vi "TempControlLoop.vi"(3 "Duty Cycle [0-100%]":dbl, 4 "Period [ms]":dbl, 5 "Count in":u32) -> (1 "State":bool, 2 "Count out":u32)   [LabVIEW 2020]
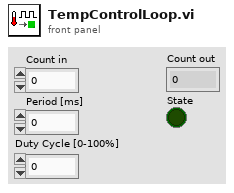
[diagram p1: front panel]
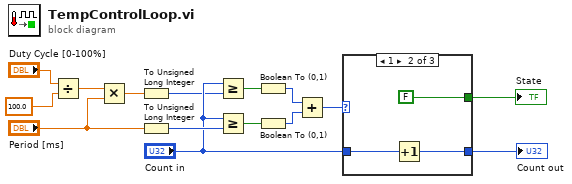
[diagram p0: block diagram]
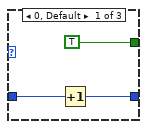
[diagram p2: hidden frame]
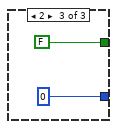
[diagram p3: hidden frame]
diagram:
  n1 = Divide(x="Duty Cycle [0-100%]", y=100.0) -> (x/y=w3:dbl)
  n2 = Multiply(x=w3, y="Period [ms]") -> (x*y=w4:dbl)
  n3 = To Unsigned Long Integer(number=w4) -> (unsigned 32bit integer=w6:u32)
  n4 = To Unsigned Long Integer(number="Period [ms]") -> (unsigned 32bit integer=w15:u32)
  n5 = Greater Or Equal?(x="Count in", y=w6) -> (x >= y?=w7:bool)
  n6 = Greater Or Equal?(x="Count in", y=w15) -> (x >= y?=w8:bool)
  n7 = Boolean To (0,1)(Boolean=w7) -> (0, 1=w9:i16)
  n8 = Boolean To (0,1)(Boolean=w8) -> (0, 1=w10:i16)
  n9 = Add(x=w9, y=w10) -> (x+y=w11:i16)
  n10 = case shown="1" w11 {
    tunnel: "Count in" -> [w18 w21 _]
    tunnel: [w17 w20 u32 0] -> w13
    tunnel: [TRUE FALSE FALSE] -> w14
    frame 0, Default {
      n11 = Increment(x=w18) -> (x+1=w17:u32)
    }
    frame 1 {
      n12 = Increment(x=w21) -> (x+1=w20:u32)
    }
    frame 2 {
    }
  }
  "State" <- w14
  "Count out" <- w13
